vi "Create Directory.vi"(8 "error in (no error)":errorcluster caption="错误输入（无错误）", 10 "Directory":path) -> (0 "error out":errorcluster caption="错误输出")   [LabVIEW 2012, in "Directory.lvclass"]
uses:
  Directory.lvclass
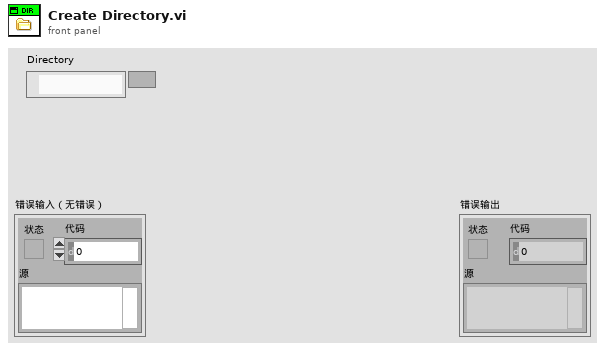
[diagram p1: front panel]
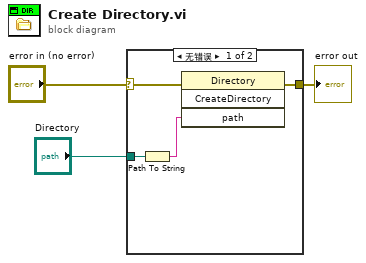
[diagram p0: block diagram]
diagram:
  n1 = case shown="无错误" "error in (no error)" {
    selector: "error in (no error)" -> [w5 w8]
    tunnel: [w4 w8] -> w2
    tunnel: "Directory" -> [w7 _]
    frame No Error {
      n2 = Path To String(path=w7) -> (string=w6:string)
      n3 = invoke on="调用节点" class="Directory" method="CreateDirectory"(error in=w5, "path"=w6) -> (error out=w4:errorcluster)  [unwired: 2 in, 3 out]
    }
    frame Error {
    }
  }
  "error out" <- w2
